vi "BRig_dataExp_T_Cue2_Audio_min.vi"() -> (2 "output_T_Cue2_Audio_min":i32)   [LabVIEW 2014]
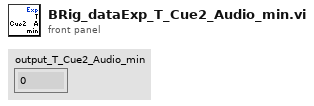
[diagram p1: front panel]
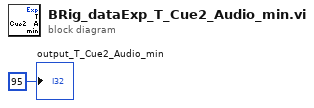
[diagram p0: block diagram]
diagram:
  "output_T_Cue2_Audio_min" <- 95 ("output_iBlock")
